vi "myRIO_BRig_FPGA_v3,71__PortC.vi"() -> ()   [LabVIEW 2014]
uses:
  <vilib>/rvi/Emulation/niFpgaGetClockAttributes.vi
  <vilib>/rvi/Emulation/niFpgaSctlEmulationGetInTimedLoop.vi
  <vilib>/rvi/Emulation/niFpgaEmulationReportErrorSimple.vi
  <vilib>/rvi/eio/common/nirviEmuTemplateMethod_errors.vi
  <vilib>/rvi/Emulation/niFpgaCriticalErrorInLSC.vi
  <vilib>/eio/EIONode/EIONode.xnode
panel:
  in  "AnaOut_1":i16
  in  "CueLed_Event":bool
  in  "CueLed_nValley":u32=100
  in  "CueLed_nPeak":u32=100
  in  "LC_Event_l2":bool
  in  "LC_Laser_l2":bool
  in  "LC_nShutter_l2":u32=100
  in  "LC_nValley_l2":u32=100
  in  "LC_nPeak_l2":u32=100
  in  "LR_wrong_nDelay_l2":u32
  in  "LR_reward_nDelay_l2":u32
  in  "LR_wrong_nTotal_l2":u32=100
  in  "LR_reward_nTotal_l2":u32=100
  in  "LR_wrong_laser_l2":bool
  in  "LR_wrong_Event_l2":bool
  in  "LR_reward_Laser_l2":bool
  in  "LR_reward_Event_l2":bool
  out "AnaIn_1":i16
  out "AnaIn_0":i16
  out "timeTrial_count":u32
  in  "timeTrial_trig":bool
  in  "k1__counter_per_ms":u16=100 min=100 max=40000 step=1
  in  "LC_nShutter_l1":u32=100
  in  "AnaOut_0":i16
  in  "LC_nValley_l1":u32=100
  in  "LC_nPeak_l1":u32=100
  in  "LC_Event_l1":bool
  in  "LR_wrong_nTotal_l1":u32=100
  in  "LR_wrong_nDelay_l1":u32
  in  "LR_reward_nTotal_l1":u32=100
  in  "LR_reward_nDelay_l1":u32
  in  "LR_reward_Event_l1":bool
  in  "LR_wrong_Event_l1":bool
  out "SelectWrong":bool
  out "SelectReward":bool
  in  "LR_wrong_Laser_l1":bool
  in  "LR_reward_Laser_l1":bool
  in  "Left(F)_or_Right(T)":bool
  in  "ignoreWrong":bool
  in  "SelectionState":bool
  in  "LC_Laser_l1":bool
  in  "FPGA_Stop":bool
  in  "audioTrigger_L":bool
  in  "audioTrigger_R":bool
  in  "audioFreq_L_kHz":u8=14 min=1 max=14 step=1
  in  "audioAmp_L":u16=1 min=1 max=32767 step=1
  in  "audioFreq_R_kHz":u8=14 min=1 max=14 step=1
  in  "audioAmp_R":u16=1 min=1 max=32767 step=1
  in  "A3_SL":bool
  in  "A1_SR":bool
  in  "Counts_Reset":bool
  out "A4_LickR":u32
  out "A2_LickL":u32
  in  "A6_Act":bool
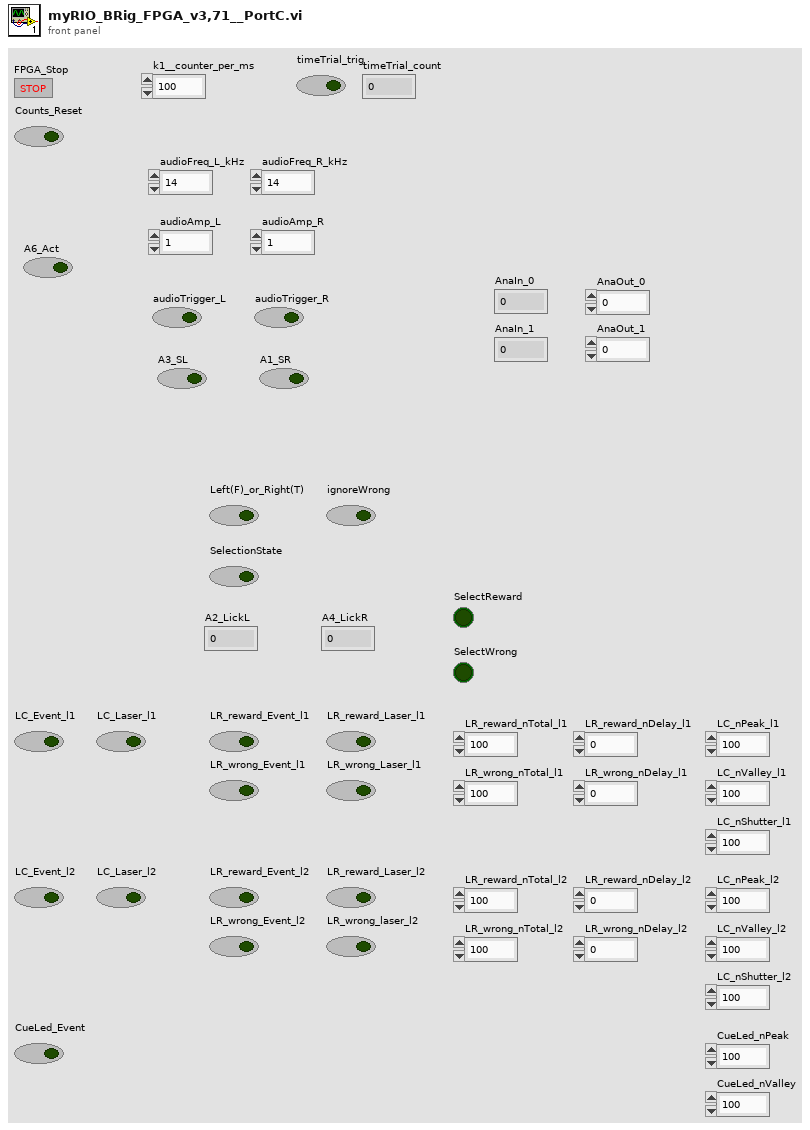
[diagram p1: front panel]
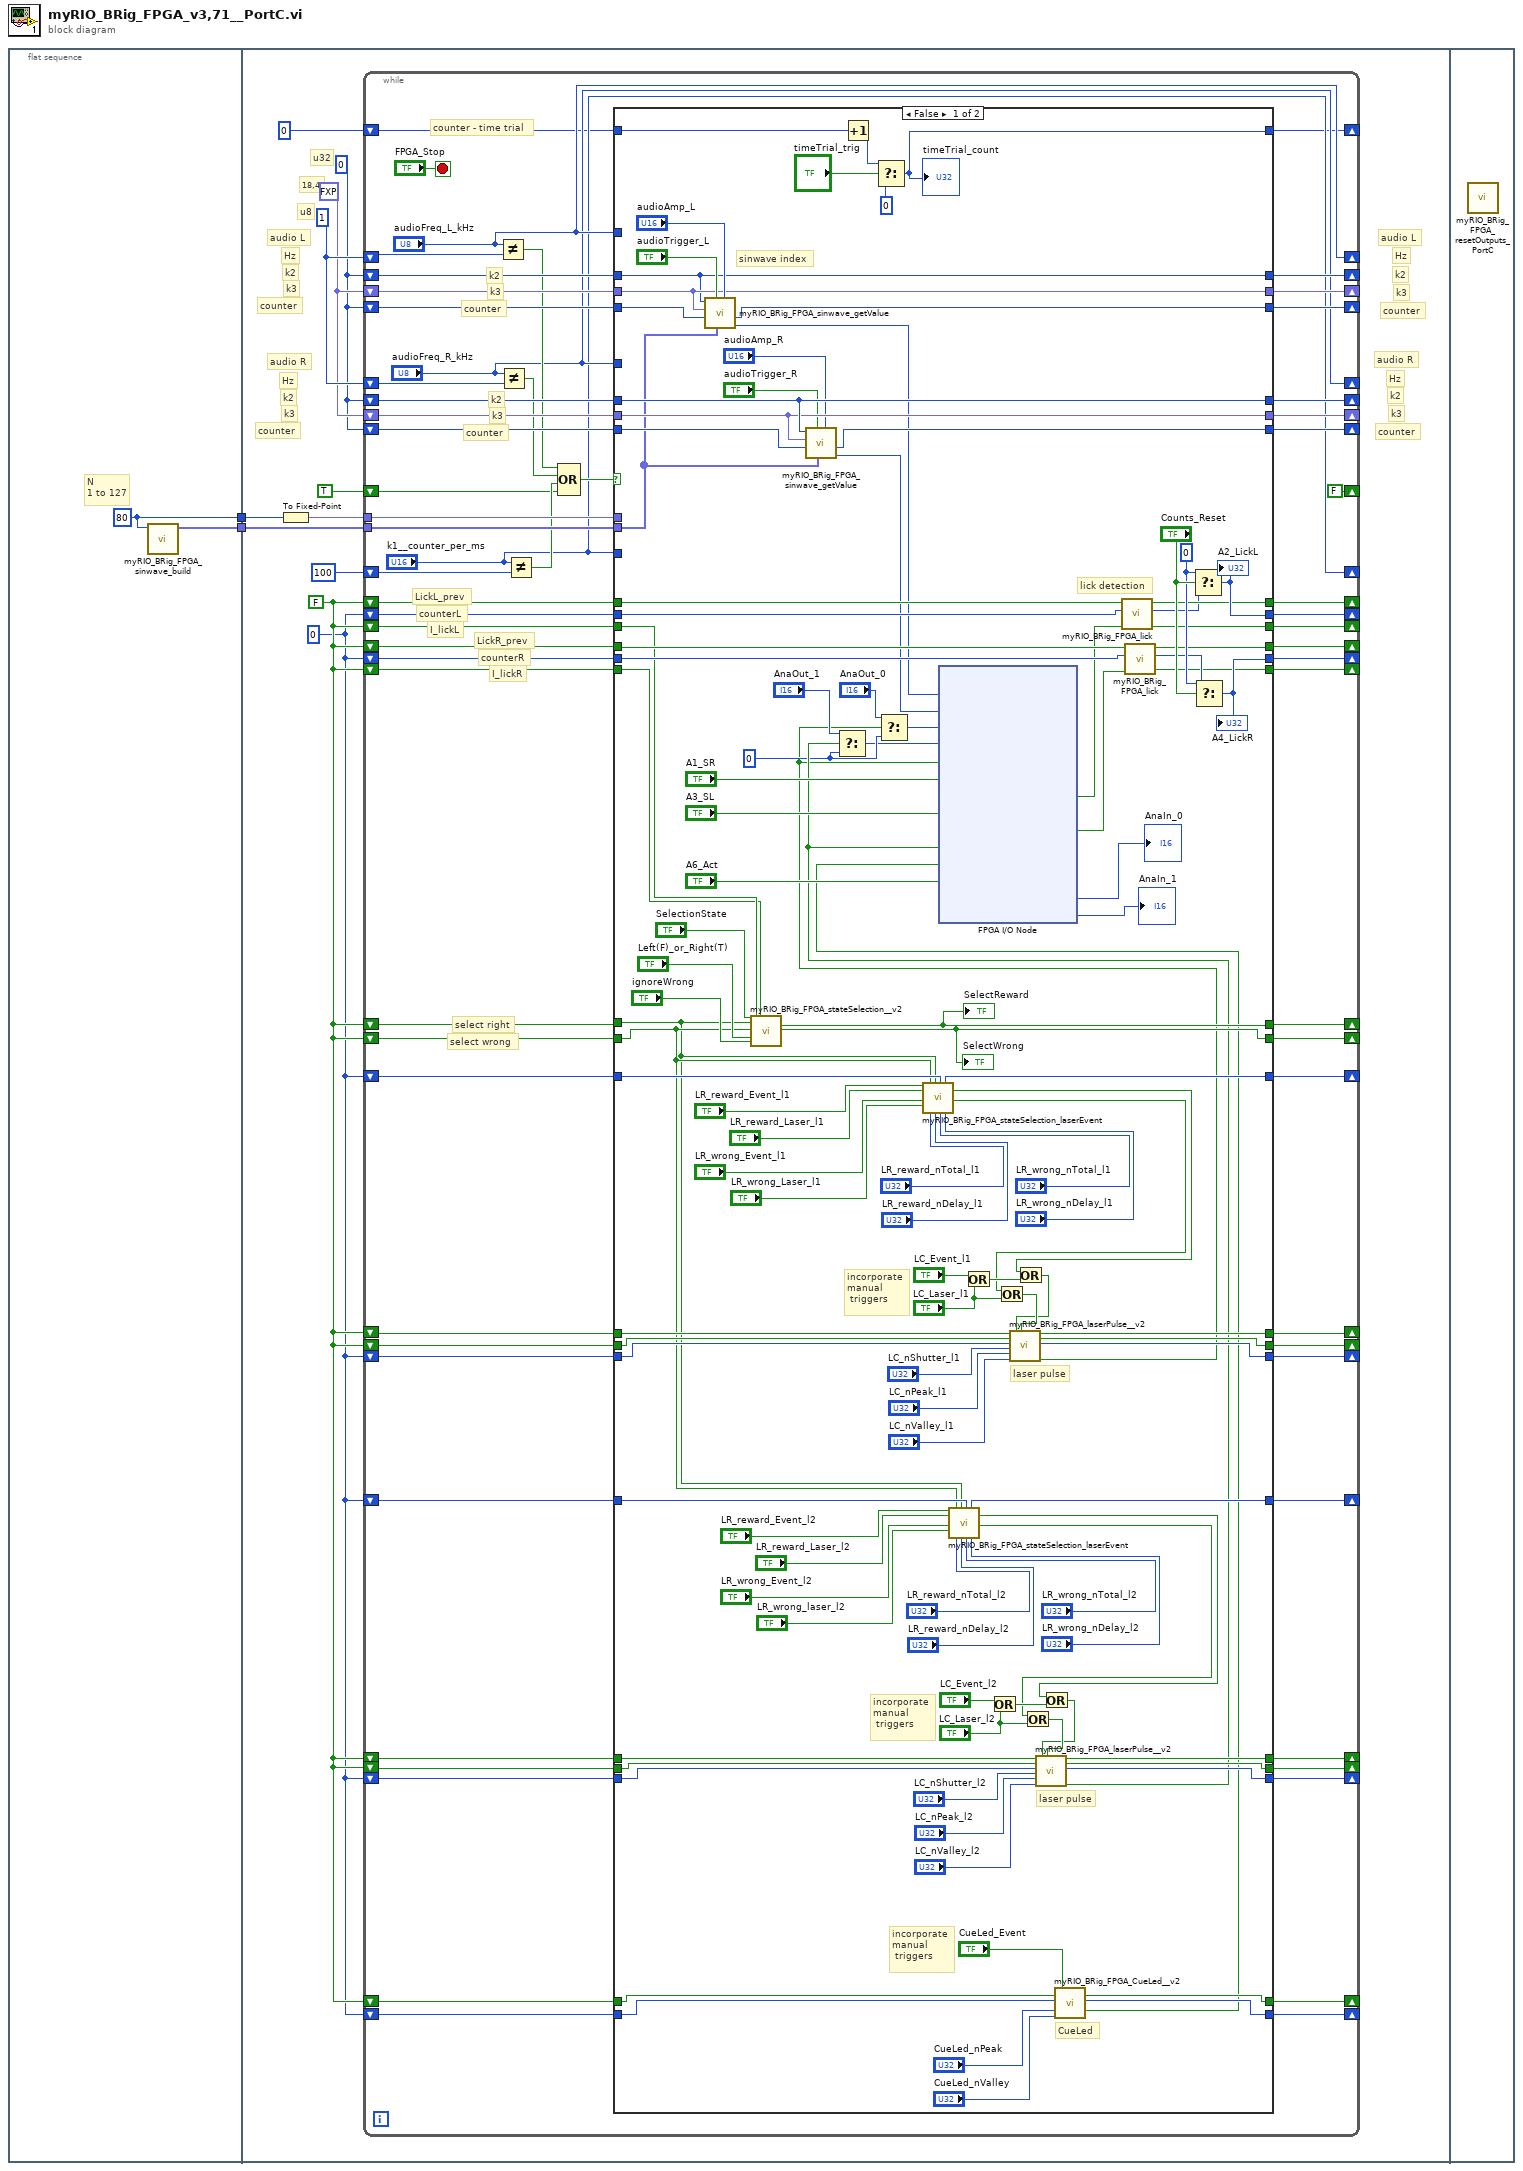
[diagram p0: block diagram]
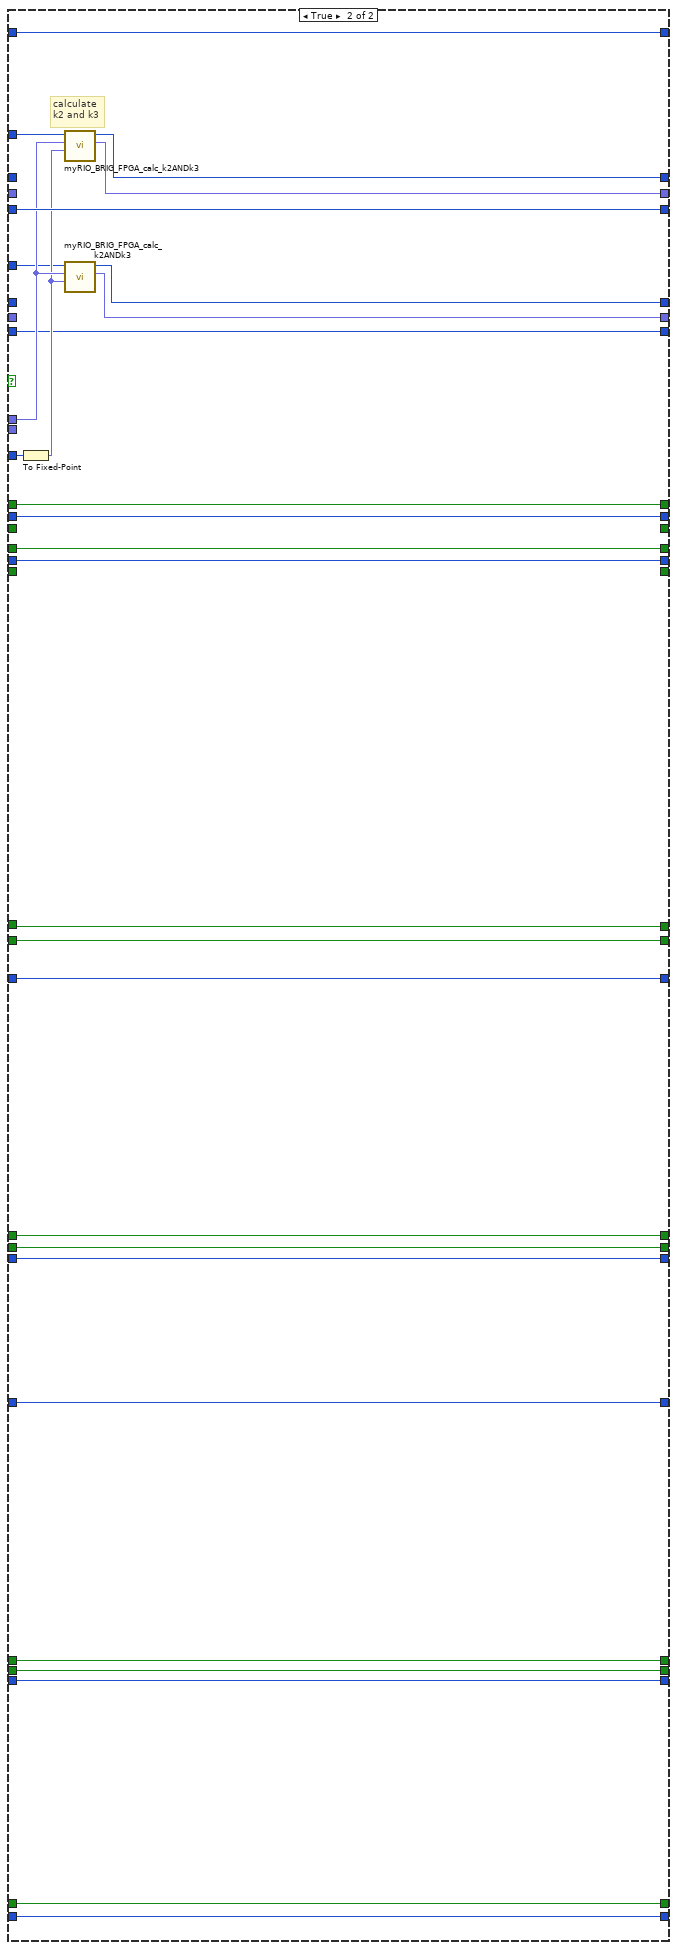
[diagram p2: hidden frame]
diagram:
  n1 = flat-sequence {
    tunnel: [w4] -> w2
    tunnel: [w3] -> w1
    tunnel: w2 -> [w15]
    tunnel: w1 -> [w14]
    frame #0 {
      w3 = 80 ("dimension size")
      # "N\n1 to 127"
      n2 = call "myRIO_BRig_FPGA_sinwave_build.vi"("input_Npts"=w3) -> ("output_array_sin"=w4:fxp<+/-,16,2>[])  [unwired: 10 in]
    }
    frame #1 {
      w5 = u32 0
      w6 = FALSE
      w10 = u32 0
      w11 = fxp<+,18,4> 0.0
      w12 = u8 1
      # "counter"
      # "k3"
      # "k2"
      # "counter"
      # "k3"
      # "k2"
      # "counter"
      # "counter"
      # "u32"
      # "k3"
      # "k2"
      # "k3"
      # "18,4"
      # "u8"
      # "Hz"
      # "Hz"
      # "audio R"
      # "audio L"
      # "Hz"
      # "k2"
      # "Hz"
      # "audio R"
      # "audio L"
      n3 = To Fixed-Point(number=w14) -> (fixed-point=w13:fxp<+,7,7>)  [unwired: 1 in]
      n4 = while {
        shift-right: ["audioFreq_L_kHz"] -> _
        shift-left: w12 -> [w80]
        shift-right: [w74] -> _
        shift-left: w10 -> [w78]
        shift-right: ["audioFreq_R_kHz"] -> _
        shift-left: w12 -> [w70]
        tunnel: w15 -> [w77]
        tunnel: w13 -> [w76]
        shift-right: [w73] -> _
        shift-left: w11 -> [w75]
        shift-right: [w71] -> _
        shift-left: w10 -> [w72]
        shift-right: [w68] -> _
        shift-left: w10 -> [w69]
        shift-right: [w66] -> _
        shift-left: w11 -> [w67]
        shift-right: [w64] -> _
        shift-left: w10 -> [w65]
        shift-right: ["k1__counter_per_ms"] -> _
        shift-left: u16 100 ("y") -> [w63]
        shift-right: [FALSE] -> _
        shift-left: TRUE -> [w58]
        shift-right: [w51] -> _
        shift-left: w6 -> [w53]
        shift-right: [w50] -> _
        shift-left: w6 -> [w52]
        shift-right: [w48] -> _
        shift-left: w5 -> [w49]
        shift-right: [w46] -> _
        shift-left: w5 -> [w47]
        shift-right: [w43] -> _
        shift-left: w6 -> [w45]
        shift-right: [w42] -> _
        shift-left: w6 -> [w44]
        shift-right: [w40] -> _
        shift-left: w6 -> [w41]
        shift-right: [w38] -> _
        shift-left: w6 -> [w39]
        shift-right: [w36] -> _
        shift-left: u32 0 -> [w37]
        shift-right: [w34] -> _
        shift-left: w5 -> [w35]
        shift-right: [w33] -> _
        shift-left: w6 -> [w30]
        shift-right: [w32] -> _
        shift-left: w6 -> [w29]
        shift-right: [w31] -> _
        shift-left: w5 -> [w28]
        shift-right: [w26] -> _
        shift-left: w5 -> [w27]
        shift-right: [w25] -> _
        shift-left: w6 -> [w22]
        shift-right: [w24] -> _
        shift-left: w6 -> [w21]
        shift-right: [w23] -> _
        shift-left: w5 -> [w20]
        shift-right: [w19] -> _
        shift-left: w6 -> [w17]
        shift-right: [w18] -> _
        shift-left: w5 -> [w16]
        stop <- "FPGA_Stop" stop-if-true
        # "counter"
        # "k3"
        # "k2"
        # "counter"
        # "k3"
        # "k2"
        # "counter - time trial"
        # "I_lickR"
        # "counterR"
        # "LickR_prev"
        # "I_lickL"
        # "counterL"
        # "LickL_prev"
        # "select wrong"
        # "select right"
        n5 = Not Equal?(x="audioFreq_L_kHz", y=w80) -> (x != y?=w62:bool)
        n6 = Not Equal?(x="audioFreq_R_kHz", y=w70) -> (x != y?=w61:bool)
        n7 = Not Equal?(x="k1__counter_per_ms", y=w63) -> (x != y?=w59:bool)
        n8 = Compound Arithmetic op=OR(w62, w61, w59, w58) -> (w60:bool)
        n9 = case shown="False" w60 {
          tunnel: w78 -> [w182 _]
          tunnel: "audioFreq_L_kHz" -> [_ w224]
          tunnel: w77 -> [w175 _]
          tunnel: w76 -> [_ w220]
          tunnel: "k1__counter_per_ms" -> [_ w225]
          tunnel: w75 -> [w183 _]
          tunnel: [w182 w223] -> w74
          tunnel: [w183 w222] -> w73
          tunnel: w72 -> [w187 w221]
          tunnel: [w184 w221] -> w71
          tunnel: w69 -> [w179 _]
          tunnel: [w179 w216] -> w68
          tunnel: w67 -> [w178 _]
          tunnel: [w178 w217] -> w66
          tunnel: w65 -> [w181 w215]
          tunnel: "audioFreq_R_kHz" -> [_ w218]
          tunnel: [w180 w215] -> w64
          tunnel: w53 -> [w170 w214]
          tunnel: w52 -> [w169 w213]
          tunnel: [w174 w214] -> w51
          tunnel: [w167 w213] -> w50
          tunnel: w49 -> [w171 w212]
          tunnel: [w197 w212] -> w48
          tunnel: w47 -> [w168 w211]
          tunnel: [w194 w211] -> w46
          tunnel: w45 -> [w102 w210]
          tunnel: w44 -> [w103 w209]
          tunnel: [w139 w210] -> w43
          tunnel: [w190 w209] -> w42
          tunnel: [w160 w206] -> w33
          tunnel: [w161 w205] -> w32
          tunnel: [w162 w204] -> w31
          tunnel: w41 -> [w164 _]
          tunnel: [w173 _] -> w40
          tunnel: w39 -> [w163 _]
          tunnel: [w165 _] -> w38
          tunnel: w37 -> [w152 w208]
          tunnel: [w149 w208] -> w36
          tunnel: w35 -> [w138 w207]
          tunnel: [w137 w207] -> w34
          tunnel: w30 -> [w128 w206]
          tunnel: w29 -> [w127 w205]
          tunnel: w28 -> [w126 w204]
          tunnel: w27 -> [w107 w203]
          tunnel: [w106 w203] -> w26
          tunnel: [w100 w202] -> w25
          tunnel: [w99 w201] -> w24
          tunnel: [w98 w200] -> w23
          tunnel: w22 -> [w97 w202]
          tunnel: w21 -> [w96 w201]
          tunnel: w20 -> [w95 w200]
          tunnel: [w92 w199] -> w19
          tunnel: [w91 w198] -> w18
          tunnel: w17 -> [w90 w199]
          tunnel: w16 -> [w89 w198]
          frame False {
            w84 = i16 0 ("f")
            w195 = u32 0 ("t")
            # "CueLed"
            # "incorporate\nmanual\n triggers"
            # "laser pulse"
            # "incorporate\nmanual\n triggers"
            # "sinwave index"
            # "lick detection"
            # "laser pulse"
            # "incorporate\nmanual\n triggers"
            n10 = call "myRIO_BRig_FPGA_sinwave_getValue.vi"("audioAmp"="audioAmp_L", "sinwave"=w175, "audioTrigger"="audioTrigger_L", "counter"=w187, "k3"=w183, "k2"=w182) -> ("output_audioValue"=w147:i16, "output_counter"=w184:u32)  [unwired: 4 in]
            n11 = call "myRIO_BRig_FPGA_stateSelection__v2.vi"("I_selectionState"="SelectionState", "I_selectRight"=w102, "I_selectWrong"=w103, "I_Left(F)_or_Right(T)"="Left(F)_or_Right(T)", "I_ignoreWrong"="ignoreWrong", "I_lickL"=w164, "I_lickR"=w163) -> ("output__I_selectRight"=w139:bool, "output__I_selectWrong"=w190:bool)  [unwired: 19 in]
            "SelectWrong" <- w190
            "SelectReward" <- w139
            n12 = call "myRIO_BRig_FPGA_sinwave_getValue.vi"("audioAmp"="audioAmp_R", "sinwave"=w175, "audioTrigger"="audioTrigger_R", "counter"=w181, "k3"=w178, "k2"=w179) -> ("output_audioValue"=w146:i16, "output_counter"=w180:u32)  [unwired: 4 in]
            n13 = Increment(x=w152) -> (x+1=w151:u32)
            n14 = Select(t=w151, s="timeTrial_trig", f=u32 0) -> (s? t:f=w149:u32)
            "timeTrial_count" <- w149
            n15 = call "myRIO_BRig_FPGA_stateSelection_laserEvent.vi"("I_LR_reward"="LR_reward_Event_l1", "I_LR_reward_laser"="LR_reward_Laser_l1", "I_LR_wrong"="LR_wrong_Event_l1", "I_LR_wrong_laser"="LR_wrong_Laser_l1", "I_selectWrong"=w103, "laser_reward_nTotal"="LR_reward_nTotal_l1", "I_selectReward"=w102, "laser_reward_nDelay"="LR_reward_nDelay_l1", "counter"=w138, "laser_wrong_nTotal"="LR_wrong_nTotal_l1", "laser_wrong_nDelay"="LR_wrong_nDelay_l1") -> ("output_counter"=w137:u32, "output_I_laserEvent"=w125:bool, "output_I_laserOn"=w124:bool)  [unwired: 6 in]
            n16 = call "myRIO_BRig_FPGA_stateSelection_laserEvent.vi"("I_LR_reward"="LR_reward_Event_l2", "I_LR_reward_laser"="LR_reward_Laser_l2", "I_LR_wrong"="LR_wrong_Event_l2", "I_LR_wrong_laser"="LR_wrong_laser_l2", "I_selectWrong"=w103, "laser_reward_nTotal"="LR_reward_nTotal_l2", "I_selectReward"=w102, "laser_reward_nDelay"="LR_reward_nDelay_l2", "counter"=w107, "laser_wrong_nTotal"="LR_wrong_nTotal_l2", "laser_wrong_nDelay"="LR_wrong_nDelay_l2") -> ("output_counter"=w106:u32, "output_I_laserEvent"=w101:bool, "output_I_laserOn"=w108:bool)  [unwired: 6 in]
            n17 = Or(x="LC_Event_l1", y="LC_Laser_l1") -> (x .or. y?=w156:bool)
            n18 = Or(x="LC_Event_l2", y="LC_Laser_l2") -> (x .or. y?=w118:bool)
            n19 = Or(x=w124, y="LC_Laser_l1") -> (x .or. y?=w154:bool)
            n20 = Or(x=w125, y=w156) -> (x .or. y?=w153:bool)
            n21 = call "myRIO_BRig_FPGA_laserPulse__v2.vi"("I_shutter"=w128, "I_peak"=w127, "count"=w126, "laser_Nshutter"="LC_nShutter_l1", "laser_Npeak"="LC_nPeak_l1", "laser_Nvalley"="LC_nValley_l1", "I_laserEvent"=w153, "I_laser"=w154) -> ("output_I_shutter"=w160:bool, "output_I_peak"=w161:bool, "output_count"=w162:u32, "output_laser"=w82:bool)  [unwired: 6 in, 2 out]
            n22 = Select(t="AnaOut_0", s=w82, f=w84) -> (s? t:f=w86:i16)
            n23 = Or(x=w108, y="LC_Laser_l2") -> (x .or. y?=w116:bool)
            n24 = Or(x=w101, y=w118) -> (x .or. y?=w115:bool)
            n25 = call "myRIO_BRig_FPGA_laserPulse__v2.vi"("I_shutter"=w97, "I_peak"=w96, "count"=w95, "laser_Nshutter"="LC_nShutter_l2", "laser_Npeak"="LC_nPeak_l2", "laser_Nvalley"="LC_nValley_l2", "I_laserEvent"=w115, "I_laser"=w116) -> ("output_I_shutter"=w100:bool, "output_I_peak"=w99:bool, "output_count"=w98:u32, "output_laser"=w85:bool)  [unwired: 6 in, 2 out]
            n26 = Select(t="AnaOut_1", s=w85, f=w84) -> (s? t:f=w81:i16)
            n27 = call "myRIO_BRig_FPGA_CueLed__v2.vi"("I_peak"=w90, "count"=w89, "laser_Npeak"="CueLed_nPeak", "laser_Nvalley"="CueLed_nValley", "I_CueLed_Event"="CueLed_Event") -> ("output_I_peak"=w92:bool, "output_count"=w91:u32, "output_led"=w88:bool)  [unwired: 12 in]
            n28 = xnode "FPGA I/O Node"("AudioOut/Left"=w147, "AudioOut/Right"=w146, "ConnectorC/AO0"=w86, "ConnectorC/AO1"=w81, "ConnectorC/DIO0"=w82, "ConnectorC/DIO1"="A1_SR", "ConnectorC/DIO3"="A3_SL", "ConnectorC/DIO5"=w85, "ConnectorC/DIO6"=w88, "ConnectorC/DIO7"="A6_Act") -> ("ConnectorC/DIO2"=w145:bool, "ConnectorC/DIO4"=w144:bool, "ConnectorC/AI0"=→"AnaIn_0":i16, "ConnectorC/AI1"=→"AnaIn_1":i16)  [unwired: 14 in, 14 out]
            n29 = call "myRIO_BRig_FPGA_lick.vi"("I_stateDetector_new"=w145, "counter"=w171, "I_stateDetector_prev"=w170) -> ("output_I_lick"=w173:bool, "output_counter"=w172:u32, "output_I_stateDetector_prev"=w174:bool)  [unwired: 6 in]
            n30 = call "myRIO_BRig_FPGA_lick.vi"("I_stateDetector_new"=w144, "counter"=w168, "I_stateDetector_prev"=w169) -> ("output_I_lick"=w165:bool, "output_counter"=w166:u32, "output_I_stateDetector_prev"=w167:bool)  [unwired: 6 in]
            n31 = Select(t=w195, s="Counts_Reset", f=w172) -> (s? t:f=w197:u32)
            "A2_LickL" <- w197
            n32 = Select(t=w195, s="Counts_Reset", f=w166) -> (s? t:f=w194:u32)
            "A4_LickR" <- w194
          }
          frame True {
            # "calculate\nk2 and k3"
            n33 = To Fixed-Point(number=w225) -> (fixed-point=w219:fxp<+,16,16>)  [unwired: 1 in]
            n34 = call "myRIO_BRIG_FPGA_calc_k2ANDk3.vi"("input_k1[count/ms]"=w219, "input_Npts"=w220, "input_freq[kHz]"=w224) -> ("output_k3"=w222:fxp<+,18,4>, "output_k2"=w223:u32)  [unwired: 7 in]
            n35 = call "myRIO_BRIG_FPGA_calc_k2ANDk3.vi"("input_k1[count/ms]"=w219, "input_Npts"=w220, "input_freq[kHz]"=w218) -> ("output_k3"=w217:fxp<+,18,4>, "output_k2"=w216:u32)  [unwired: 7 in]
          }
        }
      }
    }
    frame #2 {
      n36 = call "myRIO_BRig_FPGA_resetOutputs_PortC.vi"() -> ()  [unwired: 12 in]
    }
  }
